vi "Create ID.vi"() -> (0 "id":string)   [LabVIEW 2019, in "JSON-RPC.lvclass"]
uses:
  JSON-RPC.lvclass
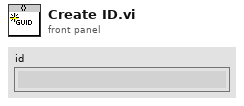
[diagram p1: front panel]
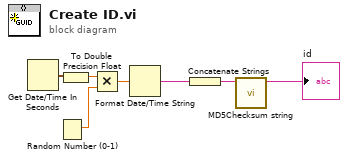
[diagram p0: block diagram]
diagram:
  n1 = Get Date/Time In Seconds() -> (seconds since 1Jan1904=w5:timestamp)
  n2 = Random Number (0-1)() -> (number: 0 to 1=w1:dbl)
  n3 = To Double Precision Float(number=w5) -> (double precision float=w6:dbl)
  n4 = Multiply(x=w6, y=w1) -> (x*y=w7:dbl)
  n5 = Format Date/Time String(seconds (now)=w7) -> (date/time string=w3:string)  [unwired: 2 in]
  n6 = Concatenate Strings(w3) -> (w2:string)
  n7 = call <vilib>:"MD5Checksum string.vi"("Message String"=w2) -> ("MD5 message-digest"=→"id":string)  [unwired: 10 in]
